vi "PathPlanner_Path_ConstTargetIncrement.vi"() -> (3 "TargetIncrement":dbl=0.05)   [LabVIEW 2019, in "PathPlanner24.lvlib"]
doc: "CONSTANT - TargetIncrement\n\nInputs: \n - <none>\n\nOutputs:\n - TargetIncrement - double -"
uses:
  PathPlanner24.lvlib
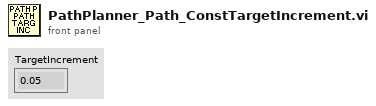
[diagram p1: front panel]
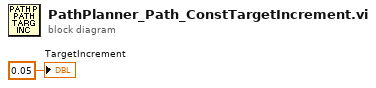
[diagram p0: block diagram]
diagram:
  "TargetIncrement" <- 0.05 ("TargetIncrement")
